vi "initialise.vi"(0 "error in (no error)":errorcluster) -> (7 "error out":errorcluster, 8 "configuration":T1, 9 "network streaming queues":T2, 10 "FPGA VI Reference Out":refnum<k20>)   [LabVIEW 2010]
uses:
  network_streaming_queues_cluster.ctl
  scan_specification_cluster.ctl
  config_data_cluster.ctl
  <vilib>/userDefined/High Color/nirio_resource_hc.ctl
  <vilib>/rvi/interface/nirviOpenFPGA/nirviOpenFPGA.xnode
  FPGA Bitfiles/PCIe-7842R_main.lvbitx
  <vilib>/rvi/ClientSDK/nirviWhatTheDeviceIsDoing.ctl
  <vilib>/rvi/interface/nirviMethod/nirviMethod.xnode
  <vilib>/rvi/interface/nirviReadWriteControl/nirviReadWriteControl.xnode
  <vilib>/rvi/interface/common/niFpgaNodeNameForErrorReporting.ctl
  <vilib>/rvi/errors/niLvFpgaWhatHappensToTopLevelVI.ctl
  <vilib>/FPGAPlugInAG/PCIe-7842R/niLvFpga_Open_PCIe-7842R.vi
  <vilib>/rvi/interface/common/dynamic/niFpgaDynamicAddResources.vi
  <vilib>/FPGAPlugInAG/Dynamic/niLvFpga_Reset_Dynamic.vi
  <vilib>/Utility/error.llb/Error Cluster From Error Code.vi
  <vilib>/rvi/errors/niLvFpgaAdjustHostInterfaceError.vi
  NiFpgaLv.dll
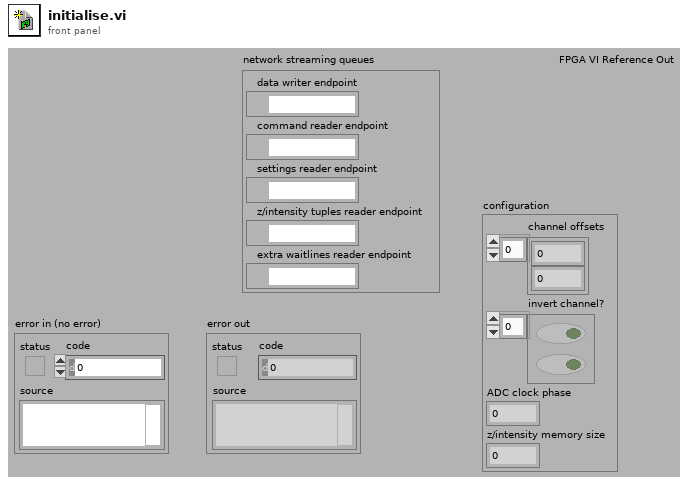
[diagram p1: front panel]
types:
  T1 = typedef "config_data_cluster.ctl" = cluster{"channel offsets":u32[], "invert channel?":bool[], "ADC clock phase":i32, "z/intensity memory size":i32}
  T2 = typedef "network_streaming_queues_cluster.ctl" = cluster{"data writer endpoint":refnum<k21>, "command reader endpoint":refnum<k21>, "settings reader endpoint":refnum<k21>, "z/intensity tuples reader endpoint":refnum<k21>, "extra waitlines reader endpoint":refnum<k21>}
  T3 = typedef "scan_specification_cluster.ctl" = cluster{"x amplitude":u16, "x resolution (pixels)":u16, "x offset fly-forward (iterations)":u16, "x offset fly-back (iterations)":u16, "y resolution (nr. of lines)":u16, "y step size":u16, "iterations per pixel":u16, "number of frames":i32, "y offset (pixels)":u16, "number of y-brake lines  (before y-fly-back)":u16, "number y-brake lines (after y-fly-back)":u16, "number of y-fly-back steps":u16, "lines per z step":u16, "number of z/intensity tuples":u16, "number of repetitions (volumes or planes)":i32, "z step size derived":u16, "choose the beginning of z scan":bool, "number of frames (settings)":i32, "FPGA trajectory?":bool}
  T4 = typedef "nirio_resource_hc.ctl" = tag
  T5 = typedef "niFpgaNodeNameForErrorReporting.ctl" = enum16{"Open FPGA VI Reference", "Read/Write Control", "Invoke Method: Abort", "Invoke Method: Acknowledge IRQ", "Invoke Method: Download", "Invoke Method: FIFO.Configure", "Invoke Method: FIFO.Read", "Invoke Method: FIFO.Start", "Invoke Method: FIFO.Stop", "Invoke Method: FIFO.Write", "Invoke Method: Reset", "Invoke Method: Run", "Invoke Method: Wait on IRQ", "Close FPGA VI Reference"}
  T6 = typedef "niLvFpgaWhatHappensToTopLevelVI.ctl" = enum16{"top level VI scripted behind XNode", "top level VI inlined behind XNode"}
  T7 = typedef "nirviWhatTheDeviceIsDoing.ctl" = enum32{"nothing", "something other than LabVIEW FPGA", "FPGA interface", "interactive", "emulation"}
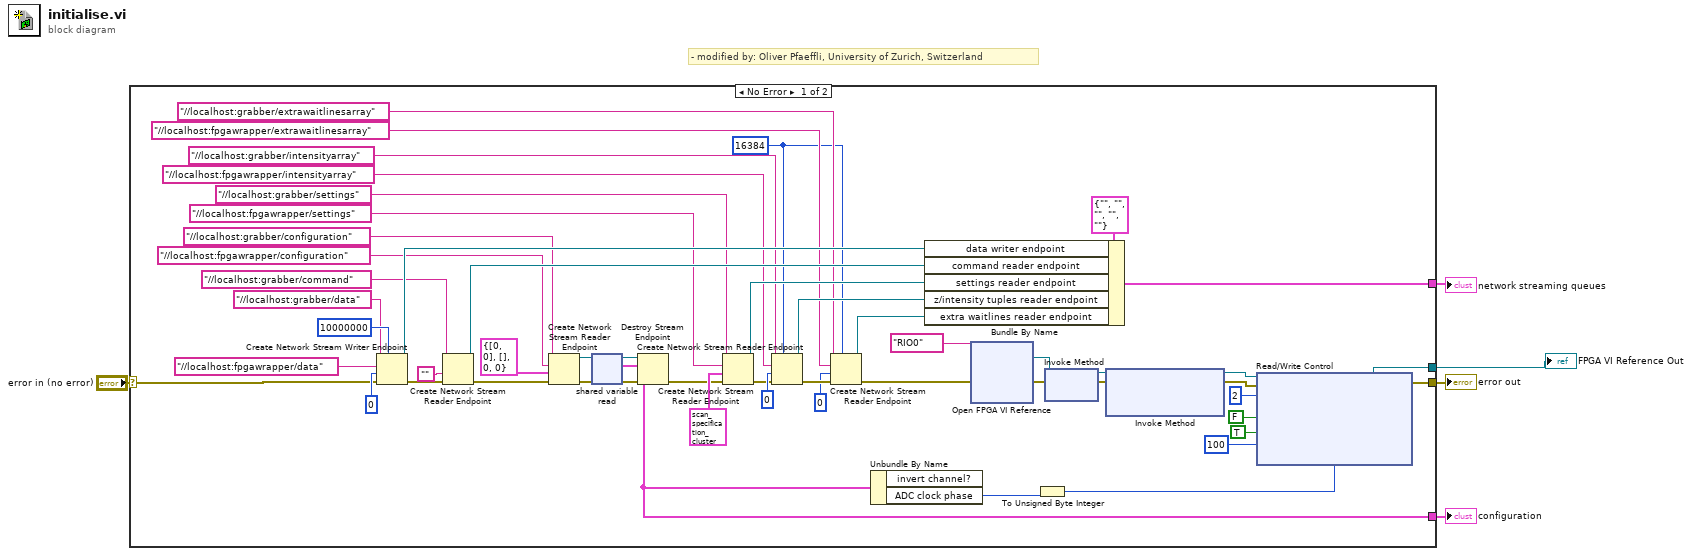
[diagram p0: block diagram]
diagram:
  # "- modified by: Oliver Pfaeffli, University of Zurich, Switzerland"
  n1 = case shown="No Error" "error in (no error)" {
    selector: "error in (no error)" -> [w29 w283]
    tunnel: [w28 w283] -> w4
    tunnel: [w49 _] -> w1
    tunnel: [w41 _] -> w3
    tunnel: [w27 _] -> w2
    frame No Error {
      w6 = 16384 ("reader buffer size")
      n2 = Create Network Stream Writer Endpoint(7:10000000 ("writer buffer size"), 8:w29, 9:u32 0, 10:"//localhost:fpgawrapper/data" ("reader url"), 11:"//localhost:grabber/data" ("writer name")) -> (0:w38:errorcluster, 3:w42:refnum<k21>)  [unwired: 1 in]
      n3 = Create Network Stream Reader Endpoint(8:w38, 9:"", 11:"//localhost:grabber/command" ("reader name")) -> (0:w13:errorcluster, 3:w37:refnum<k21>)  [unwired: 3 in]
      n4 = Create Network Stream Reader Endpoint(8:w13, 9:T1 {"channel offsets"=[0, 0], "invert channel?"=[], "ADC clock phase"=0, "z/intensity memory size"=0} ("configuration"), 10:"//localhost:fpgawrapper/configuration" ("writer name"), 11:"//localhost:grabber/configuration" ("reader name")) -> (0:w32:errorcluster, 3:w31:refnum<k21>)  [unwired: 2 in]
      n5 = shared-variable-read(w31, w32) -> (w30:refnum<k21>, w33:errorcluster, w27:T1)  [unwired: 1 in, 1 out]
      n6 = Destroy Stream Endpoint(8:w33, 11:w30) -> (0:w15:errorcluster)
      n7 = Create Network Stream Reader Endpoint(8:w15, 9:T3 {"x amplitude"=0, "x resolution (pixels)"=0, "x offset fly-forward (iterations)"=0, "x offset fly-back (iterations)"=0, "y resolution (nr. of lines)"=0, "y step size"=0, "iterations per pixel"=0, "number of frames"=0, "y offset (pixels)"=0, "number of y-brake lines  (before y-fly-back)"=0, "number y-brake lines (after y-fly-back)"=0, "number of y-fly-back steps"=0, "lines per z step"=0, "number of z/intensity tuples"=0, "number of repetitions (volumes or planes)"=0, "z step size derived"=0, "choose the beginning of z scan"=FALSE, "number of frames (settings)"=0, "FPGA trajectory?"=FALSE} ("scan specification"), 10:"//localhost:fpgawrapper/settings" ("writer name"), 11:"//localhost:grabber/settings" ("reader name")) -> (0:w14:errorcluster, 3:w20:refnum<k21>)  [unwired: 2 in]
      n8 = Create Network Stream Reader Endpoint(7:w6, 8:w14, 9:u32 0, 10:"//localhost:fpgawrapper/intensityarray" ("writer name"), 11:"//localhost:grabber/intensityarray" ("reader name")) -> (0:w12:errorcluster, 3:w16:refnum<k21>)  [unwired: 1 in]
      n9 = Create Network Stream Reader Endpoint(7:w6, 8:w12, 9:u32 0, 10:"//localhost:fpgawrapper/extrawaitlinesarray" ("writer name"), 11:"//localhost:grabber/extrawaitlinesarray" ("reader name")) -> (0:w11:errorcluster, 3:w7:refnum<k21>)  [unwired: 1 in]
      n10 = Unbundle By Name(w27) -> ("ADC clock phase"=w25:i32)  [unwired: 1 out]
      n11 = Bundle By Name(cluster=T2 {"data writer endpoint"="", "command reader endpoint"="", "settings reader endpoint"="", "z/intensity tuples reader endpoint"="", "extra waitlines reader endpoint"=""} ("network streaming queues"), "data writer endpoint"=w42, "command reader endpoint"=w37, "settings reader endpoint"=w20, "z/intensity tuples reader endpoint"=w16, "extra waitlines reader endpoint"=w7) -> (w41:T2)
      n12 = xnode "Open FPGA VI Reference"("error in"=w11, "resource name"=T4 "RIO0") -> ("FPGA VI Reference Out"=w51:refnum<k20>, "error out"=w52:errorcluster)
      n13 = To Unsigned Byte Integer(number=w25) -> (unsigned 8bit integer=w24:u8)
      n14 = xnode "Invoke Method"("FPGA VI Reference In"=w51, "error in"=w52) -> ("FPGA VI Reference Out"=w55:refnum<k20>, "error out"=w54:errorcluster)
      n15 = xnode "Invoke Method"("FPGA VI Reference In"=w55, "error in"=w54) -> ("FPGA VI Reference Out"=w57:refnum<k20>, "error out"=w56:errorcluster)  [unwired: 1 out]
      n16 = xnode "Read/Write Control"("FPGA VI Reference In"=w57, "error in"=w56, "converter box version"=i16 2, "FIFO overflow"=FALSE, "enable fly-back reversion?"=TRUE, "sync minimum high"=i16 100, "ADC clock phase"=w24) -> ("FPGA VI Reference Out"=w49:refnum<k20>, "error out"=w28:errorcluster)
    }
    frame Error {
    }
  }
  "error out" <- w4
  "network streaming queues" <- w3
  "configuration" <- w2
  "FPGA VI Reference Out" <- w1
